vi "BCU诊断标定.vi"(8 "CAN端口":u16(ring), 9 "设备索引号":u16(ring), 10 "CAN卡类型":u32(ring)=21) -> ()   [LabVIEW 2013] (continued)
              n483 = property class="Tree (严格)"(reference=w818, "Active Item Row Number"=9 ("活动项:行数"), "Disabled?"=w792, "Active Item Row Number"=1 ("活动项:行数"), "Disabled?"=w791, "Active Item Row Number"=0 ("活动项:行数"), "Disabled?"=w796, "Active Item Row Number"=3 ("活动项:行数"), "Disabled?"=w810, "Active Item Row Number"=4 ("活动项:行数"), "Disabled?"=w809, "Active Item Row Number"=5 ("活动项:行数"), "Disabled?"=w808, "Active Item Row Number"=6 ("活动项:行数"), "Disabled?"=w807, "Active Item Row Number"=7 ("活动项:行数"), "Disabled?"=w806, "Active Item Row Number"=8 ("活动项:行数"), "Disabled?"=w805, "Active Item Row Number"=11 ("活动项:行数"), "Disabled?"=w804, "Active Item Row Number"=12 ("活动项:行数"), "Disabled?"=w803, "Active Item Row Number"=13 ("活动项:行数"), "Disabled?"=w802, "Active Item Row Number"=2 ("活动项:行数"), "Disabled?"=w801, "Active Item Row Number"=10 ("活动项:行数"), "Disabled?"=w800, "Active Item Row Number"=14 ("活动项:行数"), "Disabled?"=w799) -> ()  [unwired: 1 in, 2 out]
            }
            frame #2 {
              w861 = 18
              # "一二三级故障"
              n484 = global read "功能码全局.vi" "主板故障阀值9"() -> (w867:bool[])
              n485 = Index Array(array=w867) -> (element #3=w866:bool, element #4=w863:bool, element #5=w860:bool, element #6=w865:bool, element #7=w862:bool, element #8=w859:bool)  [unwired: 8 in, 2 out]
              n486 = Not Or(1:w865, 2:w866) -> (0:w855:bool)
              n487 = Not Or(1:w862, 2:w863) -> (0:w853:bool)
              n488 = Not Or(1:w859, 2:w860) -> (0:w854:bool)
              n489 = for {
                N: w861 -> [_]
                tunnel: w856 -> [w887]
                tunnel: w855 -> [w883]
                tunnel: [w882] -> w864
                i -> [w885]
                n490 = Add(x=w885, y=15) -> (x+y=w886:i32)
                n491 = property class="Tree (严格)"(reference=w887, "Active Item Row Number"=w886, "Disabled?"=w883) -> (error out=w882:errorcluster)  [unwired: 1 in, 1 out]
              }
              n492 = for {
                N: w861 -> [_]
                tunnel: w856 -> [w881]
                tunnel: w853 -> [w877]
                tunnel: w864 -> [w876]
                tunnel: [w875] -> w858
                i -> [w879]
                n493 = Add(x=w879, y=33) -> (x+y=w880:i32)
                n494 = property class="Tree (严格)"(reference=w881, error in=w876, "Active Item Row Number"=w880, "Disabled?"=w877) -> (error out=w875:errorcluster)  [unwired: 1 out]
              }
              n495 = for {
                N: w861 -> [_]
                tunnel: w856 -> [w874]
                tunnel: w854 -> [w870]
                tunnel: w858 -> [w869]
                tunnel: [w868] -> w857
                i -> [w872]
                n496 = Add(x=w872, y=51) -> (x+y=w873:i32)
                n497 = property class="Tree (严格)"(reference=w874, error in=w869, "Active Item Row Number"=w873, "Disabled?"=w870) -> (error out=w868:errorcluster)  [unwired: 1 out]
              }
              n498 = call <vilib>:"Clear Errors.vi"("error in (no error)"=w857) -> ()  [unwired: 6 in, 1 out]
            }
          }
        }
        frame Enabled {
        }
      }
      n499 = disable-structure shown="禁用" {
        disable-tunnel: [w540 _] -> w539
        frame Disabled {
          n500 = control-ref of="从板选项"() -> (w541:refnum<vi>)
          n501 = stacked-sequence {
            tunnel: w541 -> [w544 w581 w623]
            tunnel: [w542 _ _] -> w540
            frame #0 {
              n502 = global read "功能码全局.vi" "15"() -> (w567:bool[])
              n503 = global read "功能码全局.vi" "16"() -> (w558:bool[])
              n504 = Index Array(array=w567) -> (element #1=w566:bool, element #2=w564:bool, element #3=w562:bool, element #4=w560:bool, element #5=w565:bool, element #6=w563:bool, element #7=w561:bool, element #8=w559:bool)  [unwired: 8 in]
              n505 = Index Array(array=w558) -> (element #5=w549:bool, element #6=w557:bool, element #7=w548:bool, element #8=w556:bool)  [unwired: 8 in, 4 out]
              n506 = Not Or(1:w556, 2:w557) -> (0:w546:bool)
              n507 = Not Or(1:w548, 2:w549) -> (0:w547:bool)
              n508 = Not Or(1:w565, 2:w566) -> (0:w552:bool)
              n509 = Not Or(1:w563, 2:w564) -> (0:w553:bool)
              n510 = Not Or(1:w561, 2:w562) -> (0:w554:bool)
              n511 = Not Or(1:w559, 2:w560) -> (0:w555:bool)
              n512 = Compound Arithmetic op=OR(w552, w553, w554, w555, w546) -> (w551:bool)
              "从板项目信息" <- w551
              n513 = property class="Tree (严格)"(reference=w544, "Active Item Row Number"=1 ("活动项:行数"), "Disabled?"=w551, "Active Item Row Number"=2 ("活动项:行数"), "Disabled?"=w552, "Active Item Row Number"=3 ("活动项:行数"), "Disabled?"=w553, "Active Item Row Number"=4 ("活动项:行数"), "Disabled?"=w554, "Active Item Row Number"=5 ("活动项:行数"), "Disabled?"=w555, "Active Item Row Number"=0 ("活动项:行数"), "Disabled?"=w547) -> (error out=w543:errorcluster)  [unwired: 1 in, 1 out]
              n514 = for {
                N: 8 -> [_]
                tunnel: w544 -> [w579]
                tunnel: w546 -> [w575]
                tunnel: w543 -> [w574]
                tunnel: [w573] -> w542
                i -> [w577]
                n515 = Add(x=w577, y=6) -> (x+y=w578:i32)
                n516 = property class="Tree (严格)"(reference=w579, error in=w574, "Active Item Row Number"=w578, "Disabled?"=w575) -> (error out=w573:errorcluster)  [unwired: 1 out]
              }
              n517 = call <vilib>:"Clear Errors.vi"("error in (no error)"=w542) -> ()  [unwired: 6 in, 1 out]
            }
            frame #1 {
              w592 = 8
              n518 = global read "功能码全局.vi" "18"() -> (w601:bool[])
              n519 = Index Array(array=w601) -> (element #1=w584:bool, element #2=w585:bool, element #3=w600:bool, element #4=w595:bool, element #5=w589:bool, element #6=w599:bool, element #7=w594:bool, element #8=w588:bool)  [unwired: 8 in]
              n520 = Not Or(1:w585, 2:w584) -> (0:w580:bool)
              n521 = property class="Tree (严格)"(reference=w581, "Active Item Row Number"=46 ("活动项:行数"), "Disabled?"=w580, "Active Item Row Number"=47 ("活动项:行数"), "Disabled?"=w580, "Active Item Row Number"=48 ("活动项:行数"), "Disabled?"=w580) -> ()  [unwired: 1 in, 2 out]
              n522 = Not Or(1:w588, 2:w589) -> (0:w587:bool)
              n523 = Not Or(1:w599, 2:w600) -> (0:w598:bool)
              n524 = Not Or(1:w594, 2:w595) -> (0:w593:bool)
              n525 = for {
                N: w592 -> [_]
                tunnel: w581 -> [w622]
                tunnel: w598 -> [w618]
                tunnel: "error out" -> [w617]
                tunnel: [w616] -> w596
                i -> [w620]
                n526 = Add(x=w620, y=14) -> (x+y=w621:i32)
                n527 = property class="Tree (严格)"(reference=w622, error in=w617, "Active Item Row Number"=w621, "Disabled?"=w618) -> (error out=w616:errorcluster)  [unwired: 1 out]
              }
              n528 = for {
                N: w592 -> [_]
                tunnel: w581 -> [w615]
                tunnel: w593 -> [w611]
                tunnel: w596 -> [w610]
                tunnel: [w609] -> w591
                i -> [w613]
                n529 = Add(x=w613, y=22) -> (x+y=w614:i32)
                n530 = property class="Tree (严格)"(reference=w615, error in=w610, "Active Item Row Number"=w614, "Disabled?"=w611) -> (error out=w609:errorcluster)  [unwired: 1 out]
              }
              n531 = for {
                N: w592 -> [_]
                tunnel: w581 -> [w608]
                tunnel: w587 -> [w604]
                tunnel: w591 -> [w603]
                tunnel: [w602] -> w590
                i -> [w606]
                n532 = Add(x=w606, y=30) -> (x+y=w607:i32)
                n533 = property class="Tree (严格)"(reference=w608, error in=w603, "Active Item Row Number"=w607, "Disabled?"=w604) -> (error out=w602:errorcluster)  [unwired: 1 out]
              }
              n534 = call <vilib>:"Clear Errors.vi"("error in (no error)"=w590) -> ()  [unwired: 6 in, 1 out]
            }
            frame #2 {
              n535 = global read "功能码全局.vi" "23"() -> (w647:bool[])
              n536 = global read "功能码全局.vi" "24"() -> (w645:bool[])
              n537 = Index Array(array=w647) -> (element #3=w646:bool, element #4=w643:bool, element #5=w641:bool, element #6=w639:bool, element #7=w637:bool, element #8=w635:bool)  [unwired: 8 in, 2 out]
              n538 = Index Array(array=w645) -> (element #3=w644:bool, element #4=w642:bool, element #5=w640:bool, element #6=w638:bool, element #7=w636:bool, element #8=w634:bool)  [unwired: 8 in, 2 out]
              n539 = Not Or(1:w644, 2:w646) -> (0:w633:bool)
              n540 = Not Or(1:w642, 2:w643) -> (0:w628:bool)
              n541 = Not Or(1:w640, 2:w641) -> (0:w629:bool)
              n542 = Not Or(1:w638, 2:w639) -> (0:w630:bool)
              n543 = Not Or(1:w636, 2:w637) -> (0:w632:bool)
              n544 = Not Or(1:w634, 2:w635) -> (0:w631:bool)
              n545 = Build Array(w633, w633, w632, w631, w630, w629, w628) -> (w626:bool[])
              n546 = And Array Elements(Boolean array=w626) -> (logical AND=w627:bool)
              n547 = Insert Into Array(array=w626, index=0 ("索引"), new element=w627) -> (w624:bool[])
              n548 = for {
                N: 8 -> [_]
                tunnel: w623 -> [w657]
                tunnel: w624 -> [w653] mode=indexing
                tunnel: errorcluster {"status"=FALSE, "code"=0, "source"=""} ("error out 2") -> [w652]
                tunnel: [w651] -> w649
                i -> [w655]
                n549 = Add(x=w655, y=38) -> (x+y=w656:i32)
                n550 = property class="Tree (严格)"(reference=w657, error in=w652, "Active Item Row Number"=w656, "Disabled?"=w653) -> (error out=w651:errorcluster)  [unwired: 1 out]
              }
              n551 = call <vilib>:"Clear Errors.vi"("error in (no error)"=w649) -> ()  [unwired: 6 in, 1 out]
            }
          }
        }
        frame Enabled {
        }
      }
    }
  }
  n552 = stacked-sequence {
    tunnel: w31 -> [_]
    tunnel: w34 -> [_]
    frame #0 {
    }
  }
  n553 = Obtain Queue(name (unnamed)=w43, element data type=w43, error in (no error)=w31) -> (queue out=w42:refnum<queue>, error out=w5:errorcluster)  [unwired: 2 in, 1 out]
  n554 = Obtain Queue(element data type="读参数") -> (queue out=w36:refnum<queue>, error out=w35:errorcluster)  [unwired: 4 in, 1 out]
  n555 = call <vilib>:"Open Config Data.vi"("error in (no error)"=w5, "configuration file path"=path "D:/BlueWay/BMU从板号.ini") -> ("error out"=w3:errorcluster, "refnum"=w4:T19)  [unwired: 7 in, 1 out]
  n556 = call-poly <vilib>:"Read Key.vi"("section"=w8, "error in (no error)"=w3, "default value"="BNET0001", "key"=w8, "refnum"=w4) -> ("error out"=w9:errorcluster, "value"=w1:string, "refnum out"=w10:T19)  [unwired: 3 in, 1 out]
  n557 = disable-structure shown="启用" {
    disable-tunnel: w42 -> [w895 _]
    disable-tunnel: w5 -> [w894 _]
    disable-tunnel: w34 -> [w889 _]
    disable-tunnel: w31 -> [w888 _]
    frame Enabled {
      n558 = while {
        tunnel: w895 -> [w904]
        tunnel: w894 -> [w903]
        tunnel: [w902] -> w893
        tunnel: [w901] -> w892
        tunnel: w889 -> [_]
        tunnel: w888 -> [_]
        stop <- w900 stop-if-true
        n559 = event shown="[22] \"读配置文件\": 值改变" {
          selector: _ -> [_ _ _ _ _ _ _ _ _ _ _ _ _ _ _ _ _ _ _ _ _ _ _ _ _ _ _ _ _ _ _ _ _ _ _ _ _ _ _ _ _ _ _ _ _ _ _ _ _ _ _ _ _]
          dyn-events: _ -> [_ _ _ _ _ _ _ _ _ _ _ _ _ _ _ _ _ _ _ _ _ _ _ _ _ _ _ _ _ _ _ _ _ _ _ _ _ _ _ _ _ _ _ _ _ _ _ _ _ _ _ _ _]
          timeout: 200 -> [_ _ _ _ _ _ _ _ _ _ _ _ _ _ _ _ _ _ _ _ _ _ _ _ _ _ _ _ _ _ _ _ _ _ _ _ _ _ _ _ _ _ _ _ _ _ _ _ _ _ _ _ _]
          tunnel: [_ w907 w947 _ _ _ _ _ _ _ _ _ _ _ _ _ _ _ _ _ _ _ _ _ _ _ _ _ _ _ _ _ _ _ _ _ _ _ _ _ _ _ _ _ _ _ _ _ _ _ _ _ _] -> w899
          tunnel: w904 -> [w906 w910 w946 _ w987 w998 w1009 w1020 w1031 w1042 w1053 w1064 w1075 w1086 w1097 w1108 w1124 w1647 w2059 w2084 w2112 w2215 w2288 w2301 w2311 w2357 _ _ w2407 w2474 w2541 w2608 w2675 w2742 w2809 w2877 w2945 w3012 w3079 w3149 w3160 w3199 w3239 w3279 w3319 w3357 w3417 w3452 w3488 w3521 w3591 w3624 w3657]
          tunnel: w903 -> [w905 w909 w945 _ w986 w997 w1008 w1019 w1030 w1041 w1052 w1063 w1074 w1085 w1096 w1107 w1123 w1646 w2058 w2083 w2111 w2214 w2286 w2299 w2310 w2356 _ _ w2406 w2473 w2540 w2607 w2674 w2741 w2808 w2876 w2944 w3011 w3078 w3147 w3159 w3198 w3238 w3278 w3318 w3356 w3416 w3451 w3487 w3520 w3590 w3623 w3656]
          tunnel: [w906 w910 w946 _ w987 w998 w1009 w1020 w1031 w1042 w1053 w1064 w1075 w1086 w1097 w1108 w1124 w1647 w2059 w2084 w2112 w2215 w2287 w2300 w2311 w2357 _ _ w2407 w2474 w2541 w2608 w2675 w2742 w2809 w2877 w2945 w3012 w3079 w3148 w3158 w3197 w3237 w3277 w3317 w3357 w3415 w3450 w3486 w3519 w3589 w3622 w3655] -> w902
          tunnel: [w905 w909 w945 _ w986 w997 w1008 w1019 w1030 w1041 w1052 w1063 w1074 w1085 w1096 w1107 w1123 w1646 w2058 w2083 w2111 w2214 w2285 w2298 w2310 w2356 _ _ w2406 w2473 w2540 w2607 w2674 w2741 w2808 w2876 w2944 w3011 w3078 w3146 w3157 w3196 w3236 w3276 w3316 w3356 w3414 w3449 w3485 w3518 w3588 w3621 w3654] -> w901
          tunnel: [_ _ _ _ _ _ _ _ _ _ _ _ _ _ _ _ _ _ _ _ _ _ _ _ _ _ _ _ _ _ _ _ _ _ _ _ _ _ _ _ w3157 w3196 w3236 w3276 w3316 _ w3414 w3449 w3485 w3518 w3588 w3621 w3654] -> w898
          event Timeout {
            n560 = event-data() -> ()  [unwired: 3 out]
          }
          event "停止": Value Change {
            n561 = event-data() -> ("NewVal"=w908:bool)  [unwired: 5 out]
            n562 = stacked-sequence {
              tunnel: w908 -> [w927 _]
              tunnel: [w927 _] -> w907
              frame #0 {
                n563 = global read "配置文件全局.vi" "诊断标定读取地址"() -> (w911:path)
                n564 = call <vilib>:"Application Directory.vi"() -> ("Application Directory"=w921:path)
                n565 = property class="VI"("FP.State"=T24."Hidden" ("前面板窗口:状态")) -> (reference out=w923:refnum<vi>, error out=w922:errorcluster)  [unwired: 2 in]
                n566 = Build Path(base path=w921, name or relative path="config.ini" ("名称或相对路径")) -> (appended path=w919:path)
                n567 = call <vilib>:"Open Config Data.vi"("configuration file path"=w919) -> ("error out"=w916:errorcluster, "refnum"=w918:T19)  [unwired: 8 in, 1 out]
                n568 = local write "停止"(TRUE ("停止")) -> ()
                n569 = property class="VI"(reference=w923, error in=w922, "Front Panel.Open"=FALSE ("前面板窗口:打开")) -> ()  [unwired: 2 out]
                n570 = call-poly <vilib>:"Write Key.vi"("section"="总信息", "error in (no error)"=w916, "value"=w911, "key"="诊断标定读取地址" ("section"), "refnum"=w918) -> ("error out"=w915:errorcluster, "refnum out"=w914:T19)  [unwired: 4 in, 1 out]
                n571 = call <vilib>:"Close Config Data.vi"("error in (no error)"=w915, "refnum"=w914) -> ("error out"=w913:errorcluster)  [unwired: 8 in, 1 out]
                n572 = call <vilib>:"Clear Errors.vi"("error in (no error)"=w913) -> ()  [unwired: 6 in, 1 out]
              }
              frame #1 {
                n573 = disable-structure shown="禁用" {
                  frame Disabled {
                    n574 = local read "设备索引号"() -> (w933:u16)
                    n575 = local read "CAN卡类型"() -> (w934:u32)
                    n576 = local read "CAN端口"() -> (w932:u16)
                    n577 = Build Array(7) -> (w929:i32[])
                    n578 = call "transmit-8.6.vi"("can卡类型"=w934, "设备索引号"=w933, "CAN端口"=w932, "ID"=418398080, "SendType"=u8 0, "Data"=w929) -> ()  [unwired: 3 in, 11 out]
                  }
                  frame Enabled {
                    w941 = u8 0 items=["Normal", "Listen Only"] ("工作方式")
                    w940 = u8 1 items=["Dual Filter", "Single Filter"] ("滤波方式")
                    n579 = local read "设备索引号"() -> (w936:u16)
                    n580 = local read "CAN卡类型"() -> (w935:u32)
                    n581 = local read "CAN端口"() -> (w937:u16)
                    n582 = call "CAN_Init-8.6.vi"("CAN卡类型"=w935, "设备索引号"=w936, "CAN端口"=w937, "操作类型"=enum16{"初始化CAN", "关闭CAN"}."初始化CAN", "滤波方式"=w940, "Accept Code"=u32 0, "簇"=T23 {"打开CAN"=FALSE, "初始化CAN"=TRUE, "开始CAN"=TRUE, "重启"=FALSE, "关闭CAN"=FALSE}, "Mask Code"=u32 4294967295 ("Accept Code"), "工作方式"=w941, "是否滤波"=FALSE) -> ()  [unwired: 4 in, 6 out]
                  }
                }
              }
            }
          }
          event Panel Close? {
            n583 = event-data() -> ()  [unwired: 5 out]
            n584 = stacked-sequence {
              tunnel: [w960 _] -> w947
              frame #0 {
                w960 = TRUE ("前面板窗口:打开")
                n585 = global read "配置文件全局.vi" "诊断标定读取地址"() -> (w949:path)
                n586 = call <vilib>:"Application Directory.vi"() -> ("Application Directory"=w959:path)
                n587 = property class="VI"("FP.State"=T24."Hidden" ("前面板窗口:状态")) -> (reference out=w962:refnum<vi>, error out=w961:errorcluster)  [unwired: 2 in]
                n588 = Build Path(base path=w959, name or relative path="config.ini" ("名称或相对路径")) -> (appended path=w957:path)
                n589 = call <vilib>:"Open Config Data.vi"("configuration file path"=w957) -> ("error out"=w954:errorcluster, "refnum"=w956:T19)  [unwired: 8 in, 1 out]
                n590 = property class="VI"(reference=w962, error in=w961, "Front Panel.Open"=FALSE ("前面板窗口:打开")) -> ()  [unwired: 2 out]
                n591 = call-poly <vilib>:"Write Key.vi"("section"="总信息", "error in (no error)"=w954, "value"=w949, "key"="诊断标定读取地址" ("section"), "refnum"=w956) -> ("error out"=w953:errorcluster, "refnum out"=w952:T19)  [unwired: 4 in, 1 out]
                n592 = call <vilib>:"Close Config Data.vi"("error in (no error)"=w953, "refnum"=w952) -> ("error out"=w951:errorcluster)  [unwired: 8 in, 1 out]
                n593 = call <vilib>:"Clear Errors.vi"("error in (no error)"=w951) -> ()  [unwired: 6 in, 1 out]
                n594 = local write "强制终止读写标记"(TRUE ("强制终止读写标记")) -> ()
                n595 = local write "停止"(w960) -> ()
              }
              frame #1 {
                w968 = u8 0 items=["Normal", "Listen Only"] ("工作方式")
                w969 = u8 1 items=["Dual Filter", "Single Filter"] ("滤波方式")
                n596 = local read "设备索引号"() -> (w973:u16)
                n597 = local read "CAN卡类型"() -> (w974:u32)
                n598 = local read "CAN端口"() -> (w972:u16)
                n599 = call "CAN_Init-8.6.vi"("CAN卡类型"=w974, "设备索引号"=w973, "CAN端口"=w972, "操作类型"=enum16{"初始化CAN", "关闭CAN"}."初始化CAN", "滤波方式"=w969, "Accept Code"=u32 0, "簇"=T23 {"打开CAN"=FALSE, "初始化CAN"=TRUE, "开始CAN"=TRUE, "重启"=FALSE, "关闭CAN"=FALSE}, "Mask Code"=u32 4294967295 ("Accept Code"), "工作方式"=w968, "是否滤波"=FALSE) -> ()  [unwired: 4 in, 6 out]
              }
            }
            n600 = event-data("Discard?"=w947) -> ()  [unwired: 1 in, 1 out]
          }
          event "终止读写按钮": Value Change {
            n601 = event-data() -> ("NewVal"=w975:bool)  [unwired: 6 out]
            n602 = case shown="真" w975 {
              frame False {
              }
              frame True {
                n603 = local write "强制终止读写标记"(TRUE ("强制终止读写标记")) -> ()
              }
            }
          }
          event "1": Value Change {
            w984 = FALSE ("1")
            n604 = event-data() -> ()  [unwired: 7 out]
            n605 = local write "主板2"(T8."项目信息" ("主从板")) -> ()
            n606 = Not(x=w984) -> (.not. x?=w983:bool)
            n607 = local write "1"(w983) -> ()
            n608 = local write "1 2"(w984) -> ()
            n609 = local write "1 3"(w984) -> ()
            n610 = local write "1 4"(w984) -> ()
            n611 = local write "1 5"(w984) -> ()
            n612 = local write "1 11"(w984) -> ()
            n613 = global read "功能码全局.vi" "主板监控2"() -> (w982:bool[])
            n614 = Index Array(array=w982, index=6 ("索引")) -> (element=w977:bool)
            n615 = Select(t=0, s=w977, f=1) -> (s? t:f=w978:i32)
            n616 = property on="项目信息" class="Tbl (严格)"("Disabled"=w978) -> ()  [unwired: 2 in, 2 out]
            n617 = property on="电池实际容量(A)" class="DigNum (严格)"("Disabled"=w978) -> ()  [unwired: 2 in, 2 out]
            n618 = property on="使用者" class="DigNum (严格)"("Disabled"=w978) -> ()  [unwired: 2 in, 2 out]
            n619 = property on="SOH(%)" class="DigNum (严格)"("Disabled"=w978) -> ()  [unwired: 2 in, 2 out]
            n620 = property on="电池额定容量(A)" class="DigNum (严格)"("Disabled"=w978) -> ()  [unwired: 2 in, 2 out]
            n621 = property on="SOC(%)" class="DigNum (严格)"("Disabled"=w978) -> ()  [unwired: 2 in, 2 out]
            n622 = property on="项目信息2" class="Clust (严格)"("DisabledEnum"=w978) -> ()  [unwired: 2 in, 2 out]
            n623 = property on="系统时钟" class="Str"("Disabled"=w978) -> ()  [unwired: 2 in, 2 out]
            n624 = property on="配置文件版本" class="Str"("Disabled"=w978) -> ()  [unwired: 2 in, 2 out]
            n625 = property on="车架(牌)号" class="Str"("Disabled"=w978) -> ()  [unwired: 2 in, 2 out]
            n626 = property on="产品编号" class="Str"("Disabled"=w978) -> ()  [unwired: 2 in, 2 out]
          }
          event "1 2": Value Change {
            w995 = FALSE ("1")
            n627 = event-data() -> ()  [unwired: 7 out]
            n628 = local write "主板2"(T8."一级故障阀值" ("主从板")) -> ()
            n629 = Not(x=w995) -> (.not. x?=w994:bool)
            n630 = local write "1"(w995) -> ()
            n631 = local write "1 2"(w994) -> ()
            n632 = local write "1 3"(w995) -> ()
            n633 = local write "1 4"(w995) -> ()
            n634 = local write "1 5"(w995) -> ()
            n635 = local write "1 11"(w995) -> ()
            n636 = global read "功能码全局.vi" "主板监控2"() -> (w993:bool[])
            n637 = Index Array(array=w993, index=6 ("索引")) -> (element=w988:bool)
            n638 = Select(t=0, s=w988, f=1) -> (s? t:f=w991:i32)
            n639 = property on="一级故障" class="Clust (严格)"("DisabledEnum"=w991) -> ()  [unwired: 2 in, 2 out]
          }
          event "1 3": Value Change {
            w1006 = FALSE ("1")
            n640 = event-data() -> ()  [unwired: 7 out]
            n641 = local write "主板2"(T8."二级故障阀值" ("主从板")) -> ()
            n642 = Not(x=w1006) -> (.not. x?=w1005:bool)
            n643 = local write "1"(w1006) -> ()
            n644 = local write "1 2"(w1006) -> ()
            n645 = local write "1 3"(w1005) -> ()
            n646 = local write "1 4"(w1006) -> ()
            n647 = local write "1 5"(w1006) -> ()
            n648 = local write "1 11"(w1006) -> ()
            n649 = global read "功能码全局.vi" "主板监控2"() -> (w1004:bool[])
            n650 = Index Array(array=w1004, index=6 ("索引")) -> (element=w1000:bool)
            n651 = Select(t=0, s=w1000, f=1) -> (s? t:f=w999:i32)
            n652 = property on="一级故障 2" class="Clust (严格)"("DisabledEnum"=w999) -> ()  [unwired: 2 in, 2 out]
          }
          event "1 4": Value Change {
            w1017 = FALSE ("1")
            n653 = event-data() -> ()  [unwired: 7 out]
            n654 = local write "主板2"(T8."三级故障阀值" ("主从板")) -> ()
            n655 = Not(x=w1017) -> (.not. x?=w1016:bool)
            n656 = local write "1"(w1017) -> ()
            n657 = local write "1 2"(w1017) -> ()
            n658 = local write "1 3"(w1017) -> ()
            n659 = local write "1 4"(w1016) -> ()
            n660 = local write "1 5"(w1017) -> ()
            n661 = local write "1 11"(w1017) -> ()
            n662 = global read "功能码全局.vi" "主板监控2"() -> (w1015:bool[])
            n663 = Index Array(array=w1015, index=6 ("索引")) -> (element=w1010:bool)
            n664 = Select(t=0, s=w1010, f=1) -> (s? t:f=w1013:i32)
            n665 = property on="一级故障 3" class="Clust (严格)"("DisabledEnum"=w1013) -> ()  [unwired: 2 in, 2 out]
          }
          event "1 5": Value Change {
            w1028 = FALSE ("1")
            n666 = event-data() -> ()  [unwired: 7 out]
            n667 = local write "主板2"(T8."控制参数" ("主从板")) -> ()
            n668 = Not(x=w1028) -> (.not. x?=w1027:bool)
            n669 = local write "1"(w1028) -> ()
            n670 = local write "1 2"(w1028) -> ()
            n671 = local write "1 3"(w1028) -> ()
            n672 = local write "1 4"(w1028) -> ()
            n673 = local write "1 5"(w1027) -> ()
            n674 = local write "1 11"(w1028) -> ()
            n675 = global read "功能码全局.vi" "主板监控2"() -> (w1024:bool[])
            n676 = Index Array(array=w1024, index=6 ("索引")) -> (element=w1022:bool)
            n677 = Select(t=0, s=w1022, f=1) -> (s? t:f=w1021:i32)
            n678 = property on="风机开启温度" class="DigNum (严格)"("Disabled"=w1021) -> ()  [unwired: 2 in, 2 out]
            n679 = property on="风机关闭温度" class="DigNum (严格)"("Disabled"=w1021) -> ()  [unwired: 2 in, 2 out]
            n680 = property on="加热开启温度" class="DigNum (严格)"("Disabled"=w1021) -> ()  [unwired: 2 in, 2 out]
            n681 = property on="加热关闭温度" class="DigNum (严格)"("Disabled"=w1021) -> ()  [unwired: 2 in, 2 out]
            n682 = property on="风机开启温差" class="DigNum (严格)"("Disabled"=w1021) -> ()  [unwired: 2 in, 2 out]
            n683 = property on="风机关闭温差" class="DigNum (严格)"("Disabled"=w1021) -> ()  [unwired: 2 in, 2 out]
            n684 = property on="加热控制参数" class="Clust (严格)"("DisabledEnum"=w1021) -> ()  [unwired: 2 in, 2 out]
            n685 = property on="最大允许总电压" class="DigNum (严格)"("Disabled"=w1021) -> ()  [unwired: 2 in, 2 out]
            n686 = property on="最大允许充电温度" class="DigNum (严格)"("Disabled"=w1021) -> ()  [unwired: 2 in, 2 out]
            n687 = property on="最小允许充电温度" class="DigNum (严格)"("Disabled"=w1021) -> ()  [unwired: 2 in, 2 out]
            n688 = property on="电流步长" class="DigNum (严格)"("Disabled"=w1021) -> ()  [unwired: 2 in, 2 out]
            n689 = property on="最大允许单体电压" class="DigNum (严格)"("Disabled"=w1021) -> ()  [unwired: 2 in, 2 out]
            n690 = property on="最小允许单体电压" class="DigNum (严格)"("Disabled"=w1021) -> ()  [unwired: 2 in, 2 out]
            n691 = property on="最大允许充电电流" class="DigNum (严格)"("Disabled"=w1021) -> ()  [unwired: 2 in, 2 out]
            n692 = property on="最小允许充电电流" class="DigNum (严格)"("Disabled"=w1021) -> ()  [unwired: 2 in, 2 out]
          }
          event "1 11": Value Change {
            w1039 = FALSE ("1")
            n693 = event-data() -> ()  [unwired: 7 out]
            n694 = local write "主板2"(T8."电池信息" ("主从板")) -> ()
            n695 = Not(x=w1039) -> (.not. x?=w1038:bool)
            n696 = local write "1"(w1039) -> ()
            n697 = local write "1 2"(w1039) -> ()
            n698 = local write "1 3"(w1039) -> ()
            n699 = local write "1 4"(w1039) -> ()
            n700 = local write "1 5"(w1039) -> ()
            n701 = local write "1 11"(w1038) -> ()
            n702 = global read "功能码全局.vi" "主板监控2"() -> (w1034:bool[])
            n703 = Index Array(array=w1034, index=6 ("索引")) -> (element=w1032:bool)
            n704 = Select(t=0, s=w1032, f=1) -> (s? t:f=w1035:i32)
            n705 = property on="电池串联" class="DigNum (严格)"("Disabled"=w1035) -> ()  [unwired: 2 in, 2 out]
            n706 = property on="电池并联" class="DigNum (严格)"("Disabled"=w1035) -> ()  [unwired: 2 in, 2 out]
            n707 = property on="电池包额定容量" class="DigNum (严格)"("Disabled"=w1035) -> ()  [unwired: 2 in, 2 out]
            n708 = property on="电池包额定能量(kWh)" class="DigNum (严格)"("Disabled"=w1035) -> ()  [unwired: 2 in, 2 out]
            n709 = property on="电池包额定总电压" class="DigNum (严格)"("Disabled"=w1035) -> ()  [unwired: 2 in, 2 out]
            n710 = property on="实际容量" class="DigNum (严格)"("Disabled"=w1035) -> ()  [unwired: 2 in, 2 out]
            n711 = property on="电池包组号" class="Str"("Disabled"=w1035) -> ()  [unwired: 2 in, 2 out]
            n712 = property on="电池生产日期" class="Str"("Disabled"=w1035) -> ()  [unwired: 2 in, 2 out]
            n713 = property on="电池厂家" class="Str"("Disabled"=w1035) -> ()  [unwired: 2 in, 2 out]
            n714 = property on="电池类型" class="Str"("Disabled"=w1035) -> ()  [unwired: 2 in, 2 out]
            n715 = property on="累计充电总安时" class="DigNum (严格)"("Disabled"=w1035) -> ()  [unwired: 2 in, 2 out]
            n716 = property on="累计放电总安时" class="DigNum (严格)"("Disabled"=w1035) -> ()  [unwired: 2 in, 2 out]
            n717 = property on="电池放空次数" class="DigNum (严格)"("Disabled"=w1035) -> ()  [unwired: 2 in, 2 out]
            n718 = property on="电池充满次数" class="DigNum (严格)"("Disabled"=w1035) -> ()  [unwired: 2 in, 2 out]
            n719 = property on="电池充电次数" class="DigNum (严格)"("Disabled"=w1035) -> ()  [unwired: 2 in, 2 out]
            n720 = property on="电池信息" class="Clust (严格)"("DisabledEnum"=w1035) -> ()  [unwired: 2 in, 2 out]
          }
          event "1 6": Value Change {
            w1050 = FALSE ("1 6")
            n721 = event-data() -> ()  [unwired: 7 out]
            n722 = local write "等级 2"(T21."从板信息" ("等级 2")) -> ()
            n723 = global read "功能码全局.vi" "主板监控2"() -> (w1045:bool[])
            n724 = Not(x=w1050) -> (.not. x?=w1049:bool)
            n725 = local write "1 6"(w1049) -> ()
            n726 = local write "1 7"(w1050) -> ()
            n727 = local write "1 8"(w1050) -> ()
            n728 = local write "1 9"(w1050) -> ()
            n729 = local write "1 10"(w1050) -> ()
            n730 = Index Array(array=w1045, index=6 ("索引")) -> (element=w1043:bool)
            n731 = Select(t=0, s=w1043, f=1) -> (s? t:f=w1046:i32)
            n732 = property on="项目信息 2" class="Tbl (严格)"("Disabled"=w1046) -> ()  [unwired: 2 in, 2 out]
            n733 = property on="加热控制参数" class="Clust (严格)"("Disabled"=w1046) -> ()  [unwired: 2 in, 2 out]
          }
          event "1 7": Value Change {
            w1061 = FALSE ("1 6")
            n734 = event-data() -> ()  [unwired: 7 out]
            n735 = global read "功能码全局.vi" "主板监控2"() -> (w1059:bool[])
            n736 = Index Array(array=w1059, index=6 ("索引")) -> (element=w1054:bool)
            n737 = local write "等级 2"(T21."一级故障阀值" ("等级 2")) -> ()
            n738 = Select(t=0, s=w1054, f=1) -> (s? t:f=w1055:i32)
            n739 = property on="一级故障 6" class="Clust (严格)"("DisabledEnum"=w1055) -> ()  [unwired: 2 in, 2 out]
            n740 = Not(x=w1061) -> (.not. x?=w1060:bool)
            n741 = local write "1 6"(w1061) -> ()
            n742 = local write "1 7"(w1060) -> ()
            n743 = local write "1 8"(w1061) -> ()
            n744 = local write "1 9"(w1061) -> ()
            n745 = local write "1 10"(w1061) -> ()
          }
          event "1 8": Value Change {
            w1072 = FALSE ("1 6")
            n746 = event-data() -> ()  [unwired: 7 out]
            n747 = global read "功能码全局.vi" "主板监控2"() -> (w1070:bool[])
            n748 = Index Array(array=w1070, index=6 ("索引")) -> (element=w1065:bool)
            n749 = local write "等级 2"(T21."二级故障阀值" ("等级 2")) -> ()
            n750 = Select(t=0, s=w1065, f=1) -> (s? t:f=w1066:i32)
            n751 = Not(x=w1072) -> (.not. x?=w1071:bool)
            n752 = property on="一级故障 7" class="Clust (严格)"("DisabledEnum"=w1066) -> ()  [unwired: 2 in, 2 out]
            n753 = local write "1 6"(w1072) -> ()
            n754 = local write "1 7"(w1072) -> ()
            n755 = local write "1 8"(w1071) -> ()
            n756 = local write "1 9"(w1072) -> ()
            n757 = local write "1 10"(w1072) -> ()
          }
          event "1 9": Value Change {
            w1083 = FALSE ("1 6")
            n758 = event-data() -> ()  [unwired: 7 out]
            n759 = global read "功能码全局.vi" "主板监控2"() -> (w1081:bool[])
            n760 = Index Array(array=w1081, index=6 ("索引")) -> (element=w1076:bool)
            n761 = Select(t=0, s=w1076, f=1) -> (s? t:f=w1077:i32)
            n762 = local write "等级 2"(T21."三级故障阀值" ("等级 2")) -> ()
            n763 = property on="一级故障 8" class="Clust (严格)"("DisabledEnum"=w1077) -> ()  [unwired: 2 in, 2 out]
            n764 = Not(x=w1083) -> (.not. x?=w1082:bool)
            n765 = local write "1 6"(w1083) -> ()
            n766 = local write "1 7"(w1083) -> ()
            n767 = local write "1 8"(w1083) -> ()
            n768 = local write "1 9"(w1082) -> ()
            n769 = local write "1 10"(w1083) -> ()
          }
          event "1 10": Value Change {
            w1094 = FALSE ("1 6")
            n770 = event-data() -> ()  [unwired: 7 out]
            n771 = global read "功能码全局.vi" "主板监控2"() -> (w1092:bool[])
            n772 = Index Array(array=w1092, index=6 ("索引")) -> (element=w1087:bool)
            n773 = Select(t=0, s=w1087, f=1) -> (s? t:f=w1088:i32)
            n774 = local write "等级 2"(T21."快换参数" ("等级 2")) -> ()
            n775 = property on="电池组信息" class="Clust (严格)"("Disabled"=w1088) -> ()  [unwired: 2 in, 2 out]
            n776 = Not(x=w1094) -> (.not. x?=w1093:bool)
            n777 = local write "1 6"(w1094) -> ()
            n778 = local write "1 7"(w1094) -> ()
            n779 = local write "1 8"(w1094) -> ()
            n780 = local write "1 9"(w1094) -> ()
            n781 = local write "1 10"(w1093) -> ()
          }
          event "1 12": Value Change {
            w1099 = FALSE ("1 6")
            n782 = event-data() -> ()  [unwired: 7 out]
            n783 = global read "功能码全局.vi" "主板监控2"() -> (w1106:bool[])
            n784 = Index Array(array=w1106, index=6 ("索引")) -> (element=w1102:bool)
            n785 = Select(t=0, s=w1102, f=1) -> (s? t:f=w1098:i32)
            n786 = local write "等级 2"(T14."均衡参数" ("等级 2")) -> ()
            n787 = property on="均衡参数" class="Clust (严格)"("DisabledEnum"=w1098) -> ()  [unwired: 2 in, 2 out]
            n788 = Not(x=w1099) -> (.not. x?=w1100:bool)
            n789 = local write "1 12"(w1100) -> ()
            n790 = local write "1 6"(w1099) -> ()
            n791 = local write "1 7"(w1099) -> ()
            n792 = local write "1 8"(w1099) -> ()
            n793 = local write "1 9"(w1099) -> ()
            n794 = local write "1 10"(w1099) -> ()
          }
          event "主板选项": Mouse Down {
            n795 = event-data() -> ("CtlRef"=w1122:refnum<vi>)  [unwired: 8 out]
            n796 = global read "功能码全局.vi" "主板监控2"() -> (w1111:bool[])
            n797 = property class="Tree (严格)"(reference=w1122) -> ("Value"=w1114:string)  [unwired: 1 in, 2 out]
            n798 = Index Array(array=w1111, index=6 ("索引")) -> (element=w1109:bool)
            n799 = case shown="\"温度个数\"" w1114 {
              tunnel: [T8."项目信息" ("主从板") T8."项目信息" ("主从板") T8."项目信息" ("主从板") T8."项目信息" ("主从板") T8."项目信息" ("主从板") T8."项目信息" ("主从板") T8."项目信息" ("主从板") T8."项目信息" ("主从板") T8."项目信息" ("主从板") T8."项目信息" ("主从板") T8."项目信息" ("主从板") T8."项目信息" ("主从板") T8."项目信息" ("主从板") T8."项目信息" ("主从板") T8."项目信息" ("主从板") T8."二级故障阀值" ("主从板") T8."三级故障阀值" ("主从板") T8."一级故障阀值" ("主从板") T8."控制参数" ("主从板") T8."控制参数" ("主从板") T8."电池信息" ("主从板") T8."电池信息" ("主从板") T8."电池信息" ("主从板") T8."电池信息" ("主从板") T8."电池信息" ("主从板") T8."项目信息" ("主从板")] -> w1121
              tunnel: [w1132 w1139 w1154 w1171 w1211 w1245 w1292 w1330 w1380 w1415 w1429 w1444 w1459 w1474 w1488 w1501 w1515 w1528 w1542 w1556 w1569 w1583 w1597 w1611 w1625 w1629] -> w1120
              tunnel: [w1133 w1140 w1155 w1172 w1212 w1246 w1293 w1331 w1381 w1416 w1430 w1445 w1460 w1475 w1489 w1501 w1515 w1527 w1542 w1556 w1569 w1583 w1597 w1611 w1625 w1630] -> w1119
              tunnel: [w1133 w1140 w1155 w1172 w1212 w1246 w1293 w1331 w1381 w1416 w1430 w1445 w1460 w1475 w1489 w1502 w1515 w1528 w1542 w1556 w1569 w1583 w1597 w1611 w1625 w1630] -> w1118
              tunnel: [w1133 w1140 w1155 w1172 w1212 w1246 w1293 w1331 w1381 w1416 w1430 w1445 w1460 w1475 w1489 w1501 w1514 w1528 w1542 w1556 w1569 w1583 w1597 w1611 w1625 w1630] -> w1117
              tunnel: [w1133 w1140 w1155 w1172 w1212 w1246 w1293 w1331 w1381 w1416 w1430 w1445 w1460 w1475 w1489 w1501 w1515 w1528 w1541 w1555 w1569 w1583 w1597 w1611 w1625 w1630] -> w1116
              tunnel: [w1133 w1140 w1155 w1172 w1212 w1246 w1293 w1331 w1381 w1416 w1430 w1445 w1460 w1475 w1489 w1501 w1515 w1528 w1542 w1556 w1568 w1582 w1596 w1610 w1624 w1630] -> w1115
              tunnel: [w1125 FALSE w1150 w1163 w1203 w1236 w1283 w1322 w1373 w1410 w1424 w1438 w1452 w1467 w1483 w1497 w1510 w1523 w1537 w1550 w1564 w1577 w1591 w1605 w1619 FALSE] -> w1113
              tunnel: [w1125 TRUE w1147 w1162 w1202 w1237 w1284 w1321 w1372 w1409 w1423 w1437 w1453 w1468 w1482 w1496 w1509 w1522 w1536 w1549 w1563 w1576 w1590 w1604 w1618 FALSE] -> w1112
              tunnel: w1109 -> [w1130 _ w1144 w1159 w1198 w1233 w1280 w1318 w1370 w1406 w1420 w1434 w1449 w1464 w1479 w1493 w1506 w1519 w1533 w1546 w1560 w1573 w1587 w1601 w1615 _]
              frame "项目信息" {
                w1133 = FALSE
                n800 = Select(t=0, s=w1130, f=1) -> (s? t:f=w1128:i32)
                n801 = property on="项目信息" class="Tbl (严格)"("Disabled"=w1128) -> ()  [unwired: 2 in, 2 out]
                n802 = property on="电池实际容量(A)" class="DigNum (严格)"("Disabled"=w1128) -> ()  [unwired: 2 in, 2 out]
                n803 = property on="使用者" class="DigNum (严格)"("Disabled"=w1128) -> ()  [unwired: 2 in, 2 out]
                n804 = property on="SOH(%)" class="DigNum (严格)"("Disabled"=w1128) -> ()  [unwired: 2 in, 2 out]
                n805 = property on="从板个数" class="DigNum (严格)"("NumText.BGColor"=u32 6618880) -> ()  [unwired: 2 in, 2 out]
                n806 = property on="电池额定容量(A)" class="DigNum (严格)"("Disabled"=w1128) -> ()  [unwired: 2 in, 2 out]
                n807 = property on="SOC(%)" class="DigNum (严格)"("Disabled"=w1128) -> ()  [unwired: 2 in, 2 out]
                n808 = property on="项目信息2" class="Clust (严格)"("DisabledEnum"=w1128) -> ()  [unwired: 2 in, 2 out]
                n809 = property on="系统时钟" class="Str"("Disabled"=w1128) -> ()  [unwired: 2 in, 2 out]
                n810 = property on="配置文件版本" class="Str"("Disabled"=w1128) -> ()  [unwired: 2 in, 2 out]
                n811 = property on="车架(牌)号" class="Str"("Disabled"=w1128) -> ()  [unwired: 2 in, 2 out]
                n812 = property on="产品编号" class="Str"("Disabled"=w1128) -> ()  [unwired: 2 in, 2 out]
                n813 = local read "项目信息结果"() -> (w1126:bool)
                n814 = Not(x=w1126) -> (.not. x?=w1125:bool)
                n815 = Not(x=w1133) -> (.not. x?=w1132:bool)
              }
              frame "校正时钟" {
                w1136 = 2
                w1140 = FALSE
                n816 = property on="从板个数" class="DigNum (严格)"("NumText.BGColor"=u32 13816530) -> ()  [unwired: 2 in, 2 out]
                n817 = property on="项目信息" class="Tbl (严格)"("Disabled"=w1136) -> ()  [unwired: 2 in, 2 out]
                n818 = property on="电池实际容量(A)" class="DigNum (严格)"("Disabled"=w1136) -> ()  [unwired: 2 in, 2 out]
                n819 = property on="使用者" class="DigNum (严格)"("Disabled"=w1136) -> ()  [unwired: 2 in, 2 out]
                n820 = property on="SOH(%)" class="DigNum (严格)"("Disabled"=w1136) -> ()  [unwired: 2 in, 2 out]
                n821 = property on="电池额定容量(A)" class="DigNum (严格)"("Disabled"=w1136) -> ()  [unwired: 2 in, 2 out]
                n822 = property on="SOC(%)" class="DigNum (严格)"("Disabled"=w1136) -> ()  [unwired: 2 in, 2 out]
                n823 = property on="系统时钟" class="Str"("Disabled"=w1136) -> ()  [unwired: 2 in, 2 out]
                n824 = property on="配置文件版本" class="Str"("Disabled"=w1136) -> ()  [unwired: 2 in, 2 out]
                n825 = property on="车架(牌)号" class="Str"("Disabled"=w1136) -> ()  [unwired: 2 in, 2 out]
                n826 = property on="项目信息2" class="Clust (严格)"("DisabledEnum"=w1136) -> ()  [unwired: 2 in, 2 out]
                n827 = property on="产品编号" class="Str"("Disabled"=w1136) -> ()  [unwired: 2 in, 2 out]
                n828 = Not(x=w1140) -> (.not. x?=w1139:bool)
              }
              frame "产品编号" {
                w1153 = 2
                w1155 = FALSE
                n829 = property on="项目信息" class="Tbl (严格)"("Disabled"=w1153) -> ()  [unwired: 2 in, 2 out]
                n830 = property on="电池实际容量(A)" class="DigNum (严格)"("Disabled"=w1153) -> ()  [unwired: 2 in, 2 out]
                n831 = property on="使用者" class="DigNum (严格)"("Disabled"=w1153) -> ()  [unwired: 2 in, 2 out]
                n832 = Select(t=0, s=w1144, f=1) -> (s? t:f=w1143:i32)
                n833 = property on="SOH(%)" class="DigNum (严格)"("Disabled"=w1153) -> ()  [unwired: 2 in, 2 out]
                n834 = property on="电池额定容量(A)" class="DigNum (严格)"("Disabled"=w1153) -> ()  [unwired: 2 in, 2 out]
                n835 = property on="SOC(%)" class="DigNum (严格)"("Disabled"=w1153) -> ()  [unwired: 2 in, 2 out]
                n836 = property on="产品编号" class="Str"("Disabled"=w1143) -> ()  [unwired: 2 in, 2 out]
                n837 = property on="项目信息2" class="Clust (严格)"("DisabledEnum"=w1143) -> ()  [unwired: 2 in, 2 out]
                n838 = property on="系统时钟" class="Str"("Disabled"=w1153) -> ()  [unwired: 2 in, 2 out]
                n839 = property on="配置文件版本" class="Str"("Disabled"=w1153) -> ()  [unwired: 2 in, 2 out]
                n840 = property on="车架(牌)号" class="Str"("Disabled"=w1153) -> ()  [unwired: 2 in, 2 out]
                n841 = property on="从板个数" class="DigNum (严格)"("NumText.BGColor"=u32 13816530) -> ()  [unwired: 2 in, 2 out]
                n842 = global read "功能码全局.vi" "主板项目信息5"() -> (w1151:bool[])
                n843 = global read "功能码全局.vi" "主板项目信息6"() -> (w1148:bool[])
                n844 = Index Array(array=w1151, index=0 ("索引")) -> (element=w1150:bool)
                n845 = Index Array(array=w1148, index=1 ("索引")) -> (element=w1147:bool)
                n846 = Not(x=w1155) -> (.not. x?=w1154:bool)
              }
              frame "电压个数" {
                w1170 = 2
                w1172 = FALSE
                n847 = local read "从板个数"() -> (w1169:dbl)
                n848 = property on="从板个数" class="DigNum (严格)"("NumText.BGColor"=u32 6618880) -> ()  [unwired: 2 in, 2 out]
                n849 = property on="电池实际容量(A)" class="DigNum (严格)"("Disabled"=w1170) -> ()  [unwired: 2 in, 2 out]
                n850 = property on="使用者" class="DigNum (严格)"("Disabled"=w1170) -> ()  [unwired: 2 in, 2 out]
                n851 = property on="SOH(%)" class="DigNum (严格)"("Disabled"=w1170) -> ()  [unwired: 2 in, 2 out]
                n852 = property on="电池额定容量(A)" class="DigNum (严格)"("Disabled"=w1170) -> ()  [unwired: 2 in, 2 out]
                n853 = property on="SOC(%)" class="DigNum (严格)"("Disabled"=w1170) -> ()  [unwired: 2 in, 2 out]
                n854 = property on="系统时钟" class="Str"("Disabled"=w1170) -> ()  [unwired: 2 in, 2 out]
                n855 = property on="配置文件版本" class="Str"("Disabled"=w1170) -> ()  [unwired: 2 in, 2 out]
                n856 = property on="车架(牌)号" class="Str"("Disabled"=w1170) -> ()  [unwired: 2 in, 2 out]
                n857 = property on="产品编号" class="Str"("Disabled"=w1170) -> ()  [unwired: 2 in, 2 out]
                n858 = Select(t=0, s=w1159, f=1) -> (s? t:f=w1158:i32)
                n859 = control-ref of="项目信息"() -> (w1168:refnum<vi>)
                n860 = stacked-sequence {
                  tunnel: w1169 -> [_ w1179 w1189]
                  tunnel: w1168 -> [w1174 w1178 w1190]
                  frame #0 {
                    w1175 = 0
                    n861 = Bundle(w1175, w1175) -> (w1177:cluster{i32, i32})  [unwired: 1 out]
                    n862 = property class="Tbl (严格)"(reference=w1174, "Index Values"=w1177) -> (error out=w1176:errorcluster)  [unwired: 1 in, 1 out]
                    n863 = call <vilib>:"Clear Errors.vi"("error in (no error)"=w1176) -> ()  [unwired: 7 out]
                  }
                  frame #1 {
                    n864 = for {
                      N: 10 -> [_]
                      tunnel: w1178 -> [w1188]
                      tunnel: w1179 -> [w1183]
                      i -> [w1182]
                      n865 = Compound Arithmetic op=ADD(0.0 ("值"), w1183, w1182) -> (w1185:dbl)
                      n866 = Bundle(w1185, 0) -> (w1187:cluster{dbl, i32})  [unwired: 1 out]
                      n867 = property class="Tbl (严格)"(reference=w1188, "Active Cell"=w1187, "Cell BG Color"=u32 16448250) -> ()  [unwired: 1 in, 2 out]
                    }
                  }
                  frame #2 {
                    n868 = for {
                      N: w1189 -> [_]
                      tunnel: w1190 -> [w1191]
                      i -> [w1192]
                      n869 = Bundle(w1192, 0) -> (w1196:cluster{i32, i32})  [unwired: 1 out]
                      n870 = property class="Tbl (严格)"(reference=w1191, "Active Cell"=w1196, "Cell BG Color"=u32 6618880) -> (error out=w1193:errorcluster)  [unwired: 1 in, 1 out]
                      n871 = call <vilib>:"Clear Errors.vi"("error in (no error)"=w1193) -> ()  [unwired: 7 out]
                    }
                  }
                }
                n872 = property on="项目信息" class="Tbl (严格)"("Disabled"=w1158) -> ()  [unwired: 2 in, 2 out]
                n873 = global read "功能码全局.vi" "主板项目信息5"() -> (w1166:bool[])
                n874 = global read "功能码全局.vi" "主板项目信息6"() -> (w1164:bool[])
                n875 = Index Array(array=w1166, index=1 ("索引")) -> (element=w1163:bool)
                n876 = Index Array(array=w1164, index=2 ("索引")) -> (element=w1162:bool)
                n877 = Not(x=w1172) -> (.not. x?=w1171:bool)
              }
              frame "通道电压数" {
                w1210 = 2
                w1212 = FALSE
                n878 = property on="从板个数" class="DigNum (严格)"("NumText.BGColor"=u32 13816530) -> ()  [unwired: 2 in, 2 out]
                n879 = property on="电池实际容量(A)" class="DigNum (严格)"("Disabled"=w1210) -> ()  [unwired: 2 in, 2 out]
                n880 = property on="使用者" class="DigNum (严格)"("Disabled"=w1210) -> ()  [unwired: 2 in, 2 out]
                n881 = property on="SOH(%)" class="DigNum (严格)"("Disabled"=w1210) -> ()  [unwired: 2 in, 2 out]
                n882 = property on="电池额定容量(A)" class="DigNum (严格)"("Disabled"=w1210) -> ()  [unwired: 2 in, 2 out]
                n883 = property on="SOC(%)" class="DigNum (严格)"("Disabled"=w1210) -> ()  [unwired: 2 in, 2 out]
                n884 = local read "从板个数"() -> (w1208:dbl)
                n885 = property on="系统时钟" class="Str"("Disabled"=w1210) -> ()  [unwired: 2 in, 2 out]
                n886 = property on="配置文件版本" class="Str"("Disabled"=w1210) -> ()  [unwired: 2 in, 2 out]
                n887 = property on="车架(牌)号" class="Str"("Disabled"=w1210) -> ()  [unwired: 2 in, 2 out]
                n888 = property on="产品编号" class="Str"("Disabled"=w1210) -> ()  [unwired: 2 in, 2 out]
                n889 = control-ref of="项目信息"() -> (w1209:refnum<vi>)
                n890 = stacked-sequence {
                  tunnel: w1209 -> [w1219 w1222]
                  tunnel: w1208 -> [w1218 w1221]
                  frame #0 {
                    n891 = Compound Arithmetic op=ADD(1.0 ("值"), w1218) -> (w1215:dbl)
                    n892 = Bundle(w1215, 0) -> (w1217:cluster{dbl, i32})  [unwired: 1 out]
                    n893 = property class="Tbl (严格)"(reference=w1219, "Index Values"=w1217) -> ()  [unwired: 1 in, 2 out]
                  }
                  frame #1 {
                    n894 = for {
                      N: 20 -> [_]
                      tunnel: w1222 -> [w1230]
                      tunnel: w1221 -> [w1225]
                      i -> [w1224]
                      n895 = Compound Arithmetic op=ADD(1.0 ("值"), w1225, w1224) -> (w1227:dbl)
                      n896 = Bundle(w1227, 0) -> (w1229:cluster{dbl, i32})  [unwired: 1 out]
                      n897 = property class="Tbl (严格)"(reference=w1230, "Active Cell"=w1229, "Cell BG Color"=u32 6618880) -> ()  [unwired: 1 in, 2 out]
                    }
                  }
                }
                n898 = Select(t=0, s=w1198, f=1) -> (s? t:f=w1199:i32)
                n899 = property on="项目信息" class="Tbl (严格)"("Disabled"=w1199) -> ()  [unwired: 2 in, 2 out]
                n900 = global read "功能码全局.vi" "主板项目信息5"() -> (w1206:bool[])
                n901 = global read "功能码全局.vi" "主板项目信息6"() -> (w1204:bool[])
                n902 = Index Array(array=w1206, index=2 ("索引")) -> (element=w1203:bool)
                n903 = Index Array(array=w1204, index=3 ("索引")) -> (element=w1202:bool)
                n904 = Not(x=w1212) -> (.not. x?=w1211:bool)
              }
              frame "电压起始值" {
                w1244 = 2
                w1246 = FALSE
                n905 = property on="从板个数" class="DigNum (严格)"("NumText.BGColor"=u32 13816530) -> ()  [unwired: 2 in, 2 out]
                n906 = property on="电池实际容量(A)" class="DigNum (严格)"("Disabled"=w1244) -> ()  [unwired: 2 in, 2 out]
                n907 = property on="使用者" class="DigNum (严格)"("Disabled"=w1244) -> ()  [unwired: 2 in, 2 out]
                n908 = property on="SOH(%)" class="DigNum (严格)"("Disabled"=w1244) -> ()  [unwired: 2 in, 2 out]
                n909 = property on="电池额定容量(A)" class="DigNum (严格)"("Disabled"=w1244) -> ()  [unwired: 2 in, 2 out]
                n910 = property on="SOC(%)" class="DigNum (严格)"("Disabled"=w1244) -> ()  [unwired: 2 in, 2 out]
                n911 = local read "从板个数"() -> (w1242:dbl)
                n912 = property on="系统时钟" class="Str"("Disabled"=w1244) -> ()  [unwired: 2 in, 2 out]
                n913 = property on="配置文件版本" class="Str"("Disabled"=w1244) -> ()  [unwired: 2 in, 2 out]
                n914 = property on="车架(牌)号" class="Str"("Disabled"=w1244) -> ()  [unwired: 2 in, 2 out]
                n915 = property on="产品编号" class="Str"("Disabled"=w1244) -> ()  [unwired: 2 in, 2 out]
                n916 = control-ref of="项目信息"() -> (w1243:refnum<vi>)
                n917 = stacked-sequence {
                  tunnel: w1243 -> [w1253 w1256 w1269]
                  tunnel: w1242 -> [w1252 w1255 w1268]
                  frame #0 {
                    n918 = Compound Arithmetic op=ADD(21.0 ("值"), w1252) -> (w1249:dbl)
                    n919 = Bundle(w1249, 0) -> (w1251:cluster{dbl, i32})  [unwired: 1 out]
                    n920 = property class="Tbl (严格)"(reference=w1253, "Index Values"=w1251) -> ()  [unwired: 1 in, 2 out]
                  }
                  frame #1 {
                    n921 = for {
                      N: 10 -> [_]
                      tunnel: w1256 -> [w1266]
                      tunnel: w1255 -> [w1261]
                      i -> [w1260]
                      n922 = Multiply(x=w1261, y=2.0) -> (x*y=w1258:dbl)
                      n923 = Compound Arithmetic op=ADD(21.0 ("值"), w1258, w1260) -> (w1263:dbl)
                      n924 = Bundle(w1263, 0) -> (w1265:cluster{dbl, i32})  [unwired: 1 out]
                      n925 = property class="Tbl (严格)"(reference=w1266, "Active Cell"=w1265, "Cell BG Color"=u32 16448250) -> ()  [unwired: 1 in, 2 out]
                    }
                  }
                  frame #2 {
                    n926 = Increment(x=w1268) -> (x+1=w1267:dbl)
                    n927 = for {
                      N: w1267 -> [_]
                      tunnel: w1269 -> [w1277]
                      tunnel: w1268 -> [w1272]
                      i -> [w1271]
                      n928 = Compound Arithmetic op=ADD(21.0 ("值"), w1272, w1271) -> (w1274:dbl)
                      n929 = Bundle(w1274, 0) -> (w1276:cluster{dbl, i32})  [unwired: 1 out]
                      n930 = property class="Tbl (严格)"(reference=w1277, "Active Cell"=w1276, "Cell BG Color"=u32 6618880) -> ()  [unwired: 1 in, 2 out]
                    }
                  }
                }
                n931 = Select(t=0, s=w1233, f=1) -> (s? t:f=w1232:i32)
                n932 = property on="项目信息" class="Tbl (严格)"("Disabled"=w1232) -> ()  [unwired: 2 in, 2 out]
                n933 = global read "功能码全局.vi" "主板项目信息5"() -> (w1240:bool[])
                n934 = global read "功能码全局.vi" "主板项目信息6"() -> (w1238:bool[])
                n935 = Index Array(array=w1240, index=3 ("索引")) -> (element=w1236:bool)
                n936 = Index Array(array=w1238, index=4 ("索引")) -> (element=w1237:bool)
                n937 = Not(x=w1246) -> (.not. x?=w1245:bool)
              }
              frame "温度个数" {
                w1291 = 2
                w1293 = FALSE
                n938 = property on="电池实际容量(A)" class="DigNum (严格)"("Disabled"=w1291) -> ()  [unwired: 2 in, 2 out]
                n939 = property on="使用者" class="DigNum (严格)"("Disabled"=w1291) -> ()  [unwired: 2 in, 2 out]
                n940 = property on="SOH(%)" class="DigNum (严格)"("Disabled"=w1291) -> ()  [unwired: 2 in, 2 out]
                n941 = property on="电池额定容量(A)" class="DigNum (严格)"("Disabled"=w1291) -> ()  [unwired: 2 in, 2 out]
                n942 = property on="SOC(%)" class="DigNum (严格)"("Disabled"=w1291) -> ()  [unwired: 2 in, 2 out]
                n943 = local read "从板个数"() -> (w1289:dbl)
                n944 = control-ref of="项目信息"() -> (w1290:refnum<vi>)
                n945 = stacked-sequence {
                  tunnel: w1290 -> [w1298 w1301 w1308]
                  tunnel: w1289 -> [w1295 w1300 w1307]
                  frame #0 {
                    n946 = Bundle("从板个数"=w1295, 0) -> (w1297:cluster{"从板个数":dbl, i32})  [unwired: 1 out]
                    n947 = property class="Tbl (严格)"(reference=w1298, "Index Values"=w1297) -> ()  [unwired: 1 in, 2 out]
                  }
                  frame #1 {
                    n948 = for {
                      N: 20 -> [_]
                      tunnel: w1301 -> [w1306]
                      tunnel: w1300 -> [_]
                      i -> [w1302]
                      n949 = Bundle(w1302, 0) -> (w1305:cluster{i32, i32})  [unwired: 1 out]
                      n950 = property class="Tbl (严格)"(reference=w1306, "Active Cell"=w1305, "Cell BG Color"=u32 16448250) -> ()  [unwired: 1 in, 2 out]
                    }
                  }
                  frame #2 {
                    n951 = for {
                      N: w1307 -> [_]
                      tunnel: w1308 -> [w1315]
                      tunnel: w1307 -> [w1309]
                      i -> [w1310]
                      n952 = Compound Arithmetic op=ADD(w1309, w1310) -> (w1312:dbl)
                      n953 = Bundle(w1312, 0) -> (w1314:cluster{dbl, i32})  [unwired: 1 out]
                      n954 = property class="Tbl (严格)"(reference=w1315, "Active Cell"=w1314, "Cell BG Color"=u32 6618880) -> ()  [unwired: 1 in, 2 out]
                    }
                  }
                }
                n955 = property on="系统时钟" class="Str"("Disabled"=w1291) -> ()  [unwired: 2 in, 2 out]
                n956 = property on="配置文件版本" class="Str"("Disabled"=w1291) -> ()  [unwired: 2 in, 2 out]
                n957 = property on="车架(牌)号" class="Str"("Disabled"=w1291) -> ()  [unwired: 2 in, 2 out]
                n958 = property on="产品编号" class="Str"("Disabled"=w1291) -> ()  [unwired: 2 in, 2 out]
                n959 = property on="从板个数" class="DigNum (严格)"("NumText.BGColor"=u32 13816530) -> ()  [unwired: 2 in, 2 out]
                n960 = Select(t=0, s=w1280, f=1) -> (s? t:f=w1279:i32)
